vi "Move Directory(冲突时的文件备份2013-03-27 14-07-48).vi"(7 "overwrite":bool, 8 "error in (no error)":errorcluster caption="错误输入（无错误）", 9 "NewPath":path, 10 "Path":path, 11 "FileSystem 输入":refnum<class "FileSystem.lvclass"> caption="DNL_LabVIEW Object in") -> (0 "error out":errorcluster caption="错误输出", 3 "FileSystem 输出":refnum<class "FileSystem.lvclass"> caption="DNL_LabVIEW Object out")   [LabVIEW 2012, in "FileSystem.lvclass"]
uses:
  FileSystem.lvclass
  FileSystem.lvclass/FileSystem.ctl
  Microsoft.VisualBasic
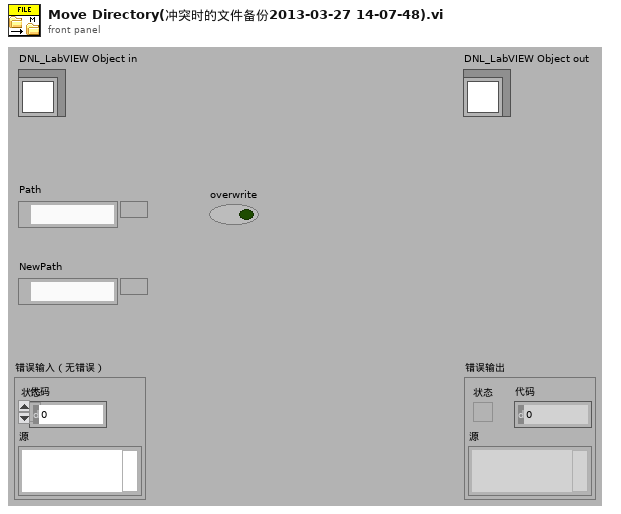
[diagram p1: front panel]
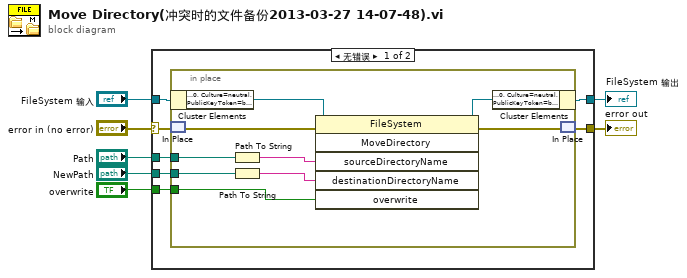
[diagram p0: block diagram]
diagram:
  n1 = case shown="无错误" "error in (no error)" {
    selector: "error in (no error)" -> [w12 w25]
    tunnel: [w11 w25] -> w6
    tunnel: [w13 w24] -> w4
    tunnel: "FileSystem 输入" -> [w14 w24]
    tunnel: "Path" -> [w10 _]
    tunnel: "NewPath" -> [w9 _]
    tunnel: "overwrite" -> [w8 _]
    frame No Error {
      n2 = in-place {
        in-place-border: w10 -> [w21]
        in-place-border: w9 -> [w17]
        in-place-border: w8 -> [w15]
        n3 = in-place-cluster #1(w14) -> ("FileSystem"=w23:refnum<k24>)
        n4 = in-place-match #2(w12) -> (w18:errorcluster)
        n5 = Path To String(path=w21) -> (string=w20:string)
        n6 = Path To String(path=w17) -> (string=w16:string)
        n7 = invoke class="FileSystem" method="MoveDirectory"(reference=w23, error in=w18, "sourceDirectoryName"=w20, "destinationDirectoryName"=w16, "overwrite"=w15) -> (reference out=w22:refnum<k24>, error out=w19:errorcluster)  [unwired: 1 in, 4 out]
        n8 = in-place-cluster #1("FileSystem"=w22) -> (w13:refnum<class "FileSystem.lvclass">)
        n9 = in-place-match #2(w19) -> (w11:errorcluster)
      }
    }
    frame Error {
    }
  }
  "error out" <- w6
  "FileSystem 输出" <- w4
